vi "Write Cancel build ref.vi"(10 "Cancel build ref":refnum<vi>, 11 "SolutionBuilder in":refnum<class "SolutionBuilder.lvclass">) -> (3 "SolutionBuilder out":refnum<class "SolutionBuilder.lvclass">)   [LabVIEW 2019, in "SolutionBuilder.lvlib" / "SolutionBuilder.lvclass"]
uses:
  SolutionBuilder.lvclass
  SolutionBuilder.lvclass/SolutionBuilder.ctl
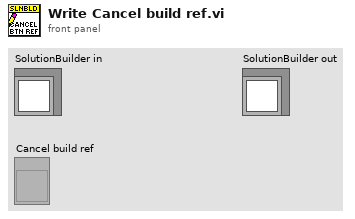
[diagram p1: front panel]
types:
  T1 = enum8{"Enabled", "Disabled", "Disabled and Grayed Out"}
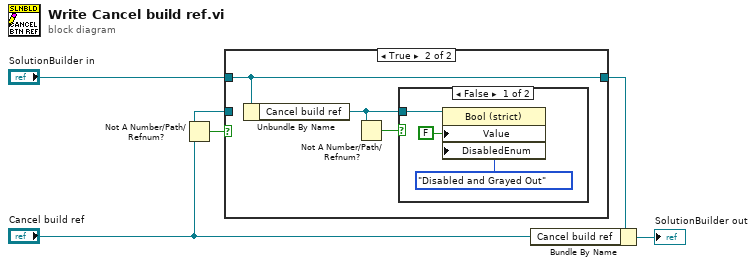
[diagram p0: block diagram]
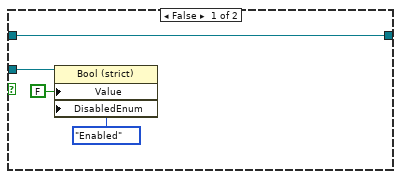
[diagram p2: hidden frame]
diagram:
  n1 = Not A Number/Path/Refnum?(number/path/refnum="Cancel build ref") -> (NaN/Path/Refnum?=w4:bool)
  n2 = case shown="True" w4 {
    tunnel: "SolutionBuilder in" -> [w8 w12]
    tunnel: [w8 w12] -> w2
    tunnel: "Cancel build ref" -> [w7 _]
    frame False {
      n3 = property class="Bool (strict)"(reference=w7, "Value"=FALSE, "DisabledEnum"=T1."Enabled" ("Disabled")) -> ()  [unwired: 1 in, 2 out]
    }
    frame True {
      n4 = Unbundle By Name(w12) -> ("Cancel build ref"=w10:refnum<vi>)
      n5 = Not A Number/Path/Refnum?(number/path/refnum=w10) -> (NaN/Path/Refnum?=w11:bool)
      n6 = case shown="False" w11 {
        tunnel: w10 -> [w15 _]
        frame False {
          n7 = property class="Bool (strict)"(reference=w15, "Value"=FALSE, "DisabledEnum"=T1."Disabled and Grayed Out" ("Disabled")) -> ()  [unwired: 1 in, 2 out]
        }
        frame True {
        }
      }
    }
  }
  n8 = Bundle By Name(cluster=w2, "Cancel build ref"="Cancel build ref") -> (→"SolutionBuilder out":refnum<class "SolutionBuilder.lvclass">)
